vi "Backpressure - unbounded no loss.vi"(8 "error in (no error)":errorcluster) -> (0 "error out":errorcluster)   [LabVIEW 2026, in "Tests.lvlib"]
doc: "Integration test. Verifies that a single Log call fans out to every registered appender: registers three queue-mode relay appenders, logs one Info message, and asserts each appender's queue receives exactly one Statement with identical payload. Every gate except fan-out is held open (global threshold at floor, permissive filters, unbounded queues), so a missing element can only be a fan-out defect.\n\nImplements LMBR-T-030 -> SRS-019, SRS-028. Assert-level IDs: Test-ID-Assert-Checklist.md."
uses:
  Tests.lvlib
  src/TypeDefs/Severity.ctl
  <vilib>/addons/_JKI Toolkits/Caraya/classes/Assert/Assert Equal Value_Variant.vi
  <vilib>/addons/_JKI Toolkits/Caraya/classes/Test/Test.lvclass
  src/Lumberjack.lvlib
  src/Public/Logger.lvclass/Logger.lvclass
  <vilib>/addons/_JKI Toolkits/Caraya/classes/Assert/Assert.lvclass
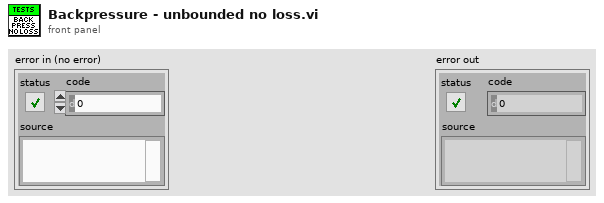
[diagram p1: front panel]
types:
  T1 = typedef "Lumberjack.lvlib/Severity.ctl" = enum16{"OFF", "FATAL", "ERROR", "WARN", "INFO", "DEBUG", "TRACE", "ALL"}
  T2 = typedef "Lumberjack.lvlib/Statement.ctl" = cluster{"timestamp":timestamp, "level":T1, "sourceTag":string, "originVI":string, "message":string}
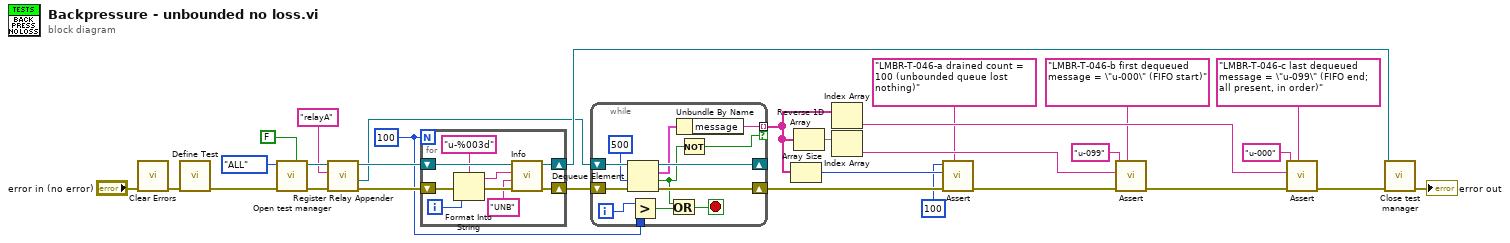
[diagram p0: block diagram]
diagram:
  w3 = 100
  n1 = call <vilib>:"Clear Errors.vi"("error in (no error)"="error in (no error)") -> ("error out"=w1:errorcluster)  [unwired: 5 in, 1 out]
  n2 = call <vilib>:"Define Test.vi"("error in (no error)"=w1) -> ("error out"=w30:errorcluster)  [unwired: 9 in, 1 out]
  n3 = call "Open test manager.vi"("enableDefaultFile"=FALSE, "error in (no error)"=w30, "globalThreshold"=Severity."ALL") -> ("error out"=w24:errorcluster, "Logger out"=w25:refnum<class "Logger.lvclass">)  [unwired: 7 in]
  n4 = call "Register Relay Appender.vi"("error in (no error)"=w24, "id in"="relayA", "Logger in"=w25) -> ("error out"=w22:errorcluster, "relayQueue"=w21:refnum<queue>, "Logger out"=w23:refnum<class "Logger.lvclass">)  [unwired: 5 in, 1 out]
  n5 = for {
    N: w3 -> [_]
    shift-right: [w38] -> w26
    shift-left: w23 -> [w37]
    shift-right: [w39] -> w28
    shift-left: w22 -> [w36]
    i -> [w31]
    n6 = Format Into String(format string="u-%003d" ("message"), error in=w36, w31) -> (resulting string=w33:string, error out=w35:errorcluster)  [unwired: 1 in]
    n7 = call "Info.vi"("error in (no error)"=w35, "sourceTag"="UNB", "message"=w33, "Logger in"=w37) -> ("error out"=w39:errorcluster, "Logger out"=w38:refnum<class "Logger.lvclass">)  [unwired: 6 in]
  }
  n8 = while {
    shift-right: [w47] -> w18
    shift-left: w28 -> [w52]
    shift-right: [w49] -> _
    shift-left: w21 -> [w51]
    tunnel: [w46] -> w15 mode=indexing if=w45
    tunnel: w3 -> [w43]
    i -> [w44]
    stop <- w40 stop-if-true
    n9 = Dequeue Element(queue=w51, timeout in ms (-1)=500, error in (no error)=w52) -> (queue out=w49:refnum<queue>, element=w48:T2, timed out?=w41:bool, error out=w47:errorcluster)
    n10 = Greater?(x=w44, y=w43) -> (0:w42:bool)
    n11 = Or(x=w41, y=w42) -> (x .or. y?=w40:bool)
    n12 = Unbundle By Name(w48) -> ("message"=w46:string)
    n13 = Not(x=w41) -> (.not. x?=w45:bool)
  }
  n14 = Array Size(array=w15) -> (size(s)=w17:i32)
  n15 = Reverse 1D Array(array=w15) -> (reversed array=w14:string[])
  n16 = Index Array(array=w15) -> (element=w10:string)  [unwired: 1 in]
  n17 = Index Array(array=w14) -> (element=w9:string)  [unwired: 1 in]
  n18 = call-poly <vilib>:"Assert.vi"("Label"="LMBR-T-046-a drained count = 100 (unbounded queue lost nothing)", "error in (no error)"=w18, "Actual"=w17, "Expected"=100 ("size(s)")) -> ("error out"=w13:errorcluster)  [unwired: 6 in, 1 out]
  n19 = call-poly <vilib>:"Assert.vi"("Label"="LMBR-T-046-b first dequeued message = \"u-000\" (FIFO start)", "error in (no error)"=w13, "Actual"=w9, "Expected"="u-099") -> ("error out"=w12:errorcluster)  [unwired: 6 in, 1 out]
  n20 = call-poly <vilib>:"Assert.vi"("Label"="LMBR-T-046-c last dequeued message = \"u-099\" (FIFO end; all present, in order)", "error in (no error)"=w12, "Actual"=w10, "Expected"="u-000") -> ("error out"=w11:errorcluster)  [unwired: 6 in, 1 out]
  n21 = call "Close test manager.vi"("error in (no error)"=w11, "Logger in"=w26) -> ("error out"=→"error out":errorcluster)  [unwired: 7 in]
